vi "PlotCache.vi"(8 "Op":T1(ring), 9 "PlotName":string, 11 "Plot":cluster{"Days":timestamp[], dbl[]}[](graph)) -> (0 "Name":string, 2 "Names":string[](array[string]), 3 "PlotOut":cluster{"Days":timestamp[], dbl[]}[](graph))   [LabVIEW 2017]
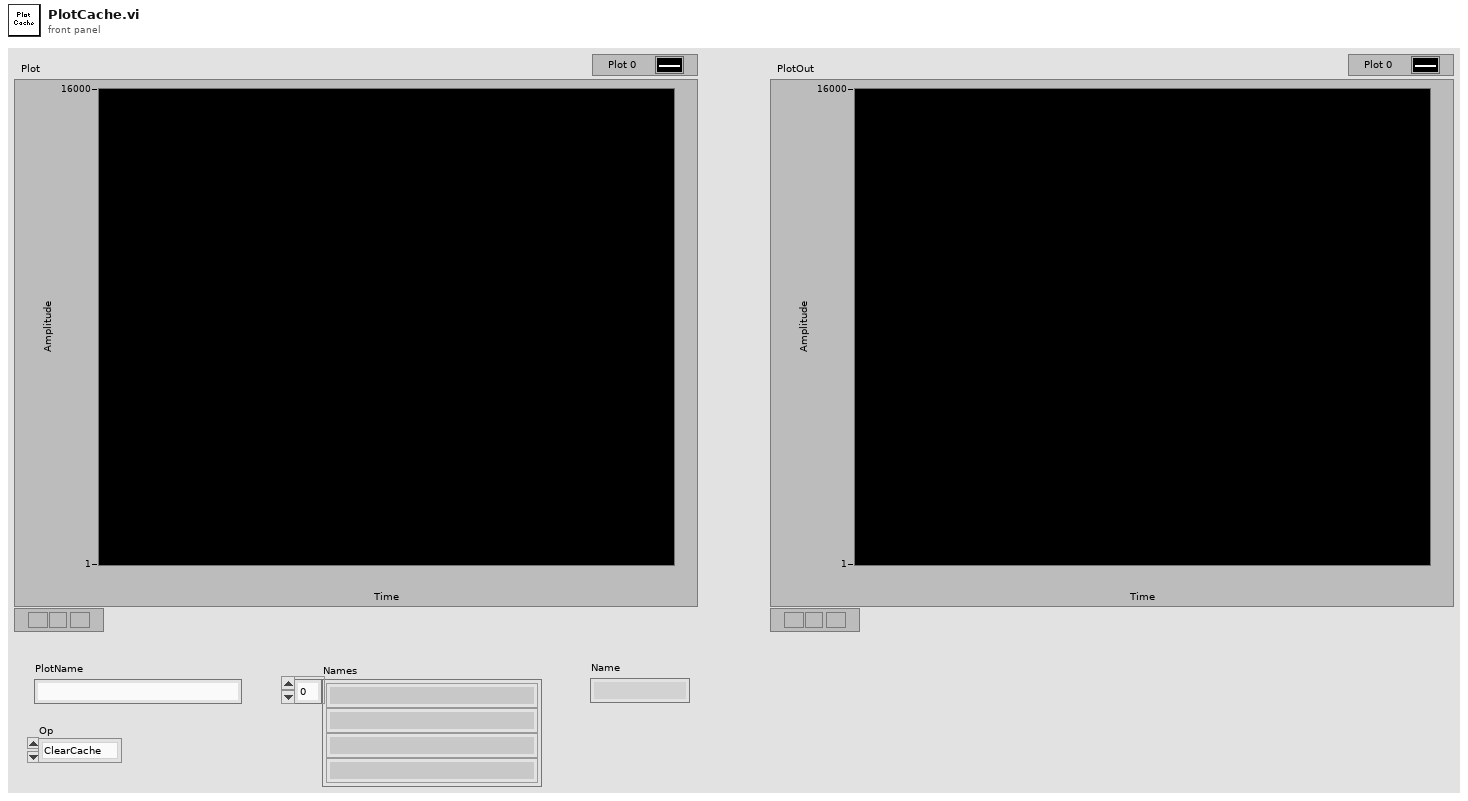
[diagram p1: front panel]
types:
  T1 = enum16{"ClearCache", "AddPlot", "GetPlot", "GetNames", "LastPlot"}
  T2 = cluster{"PlotName":string, "Plot":cluster{"Days":timestamp[], dbl[]}[]}[]
  T3 = cluster{"PlotName":string, "Plot":cluster{"Days":timestamp[], dbl[]}[]}
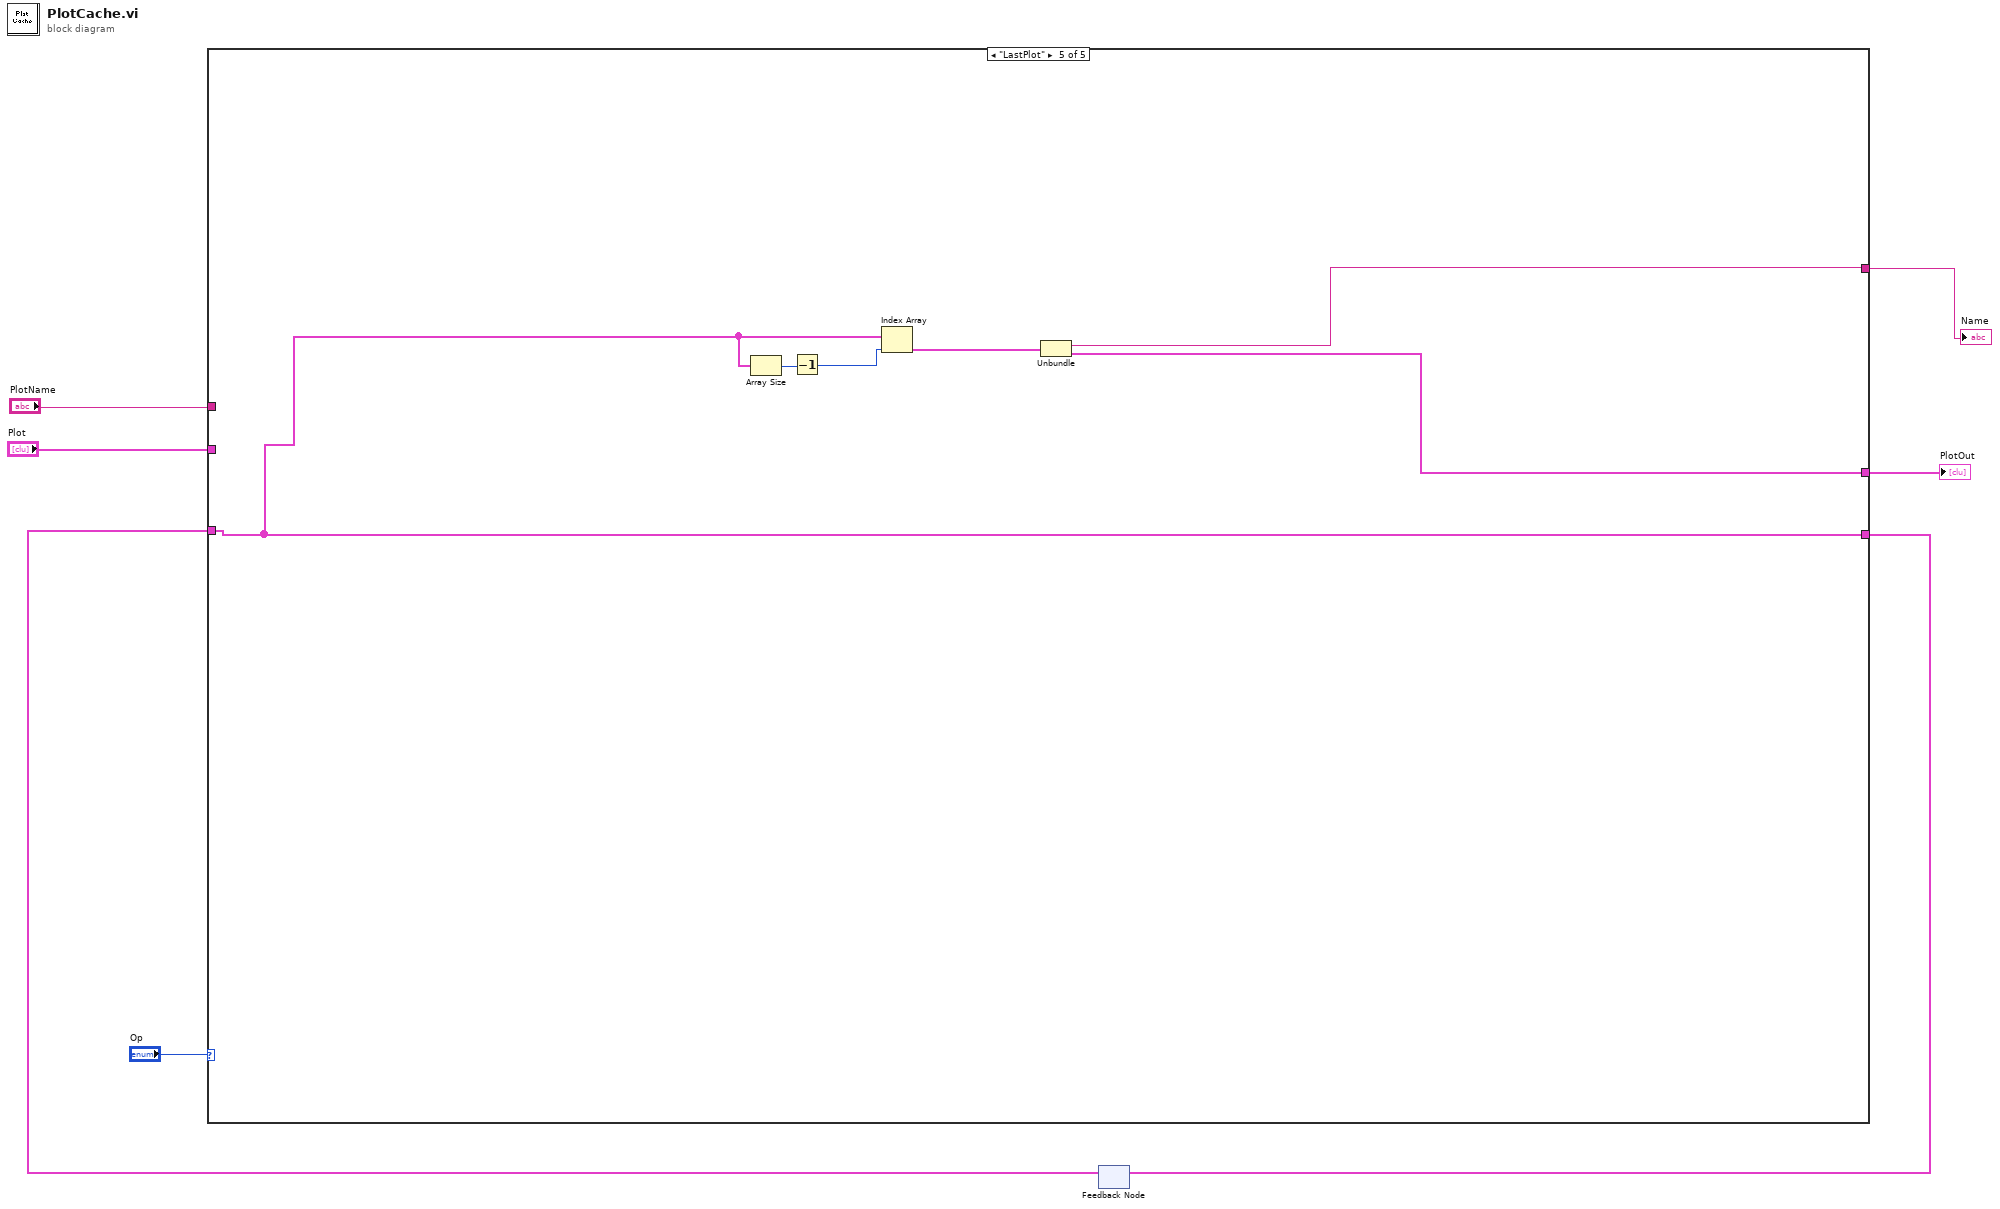
[diagram p0: block diagram]
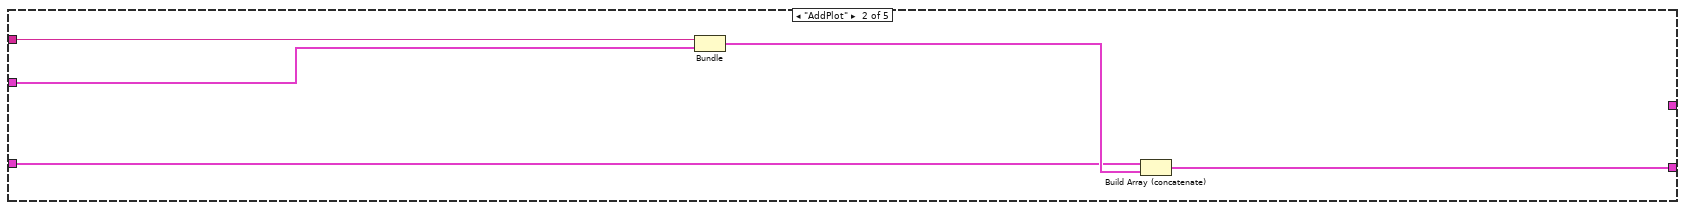
[diagram p3: hidden frame]
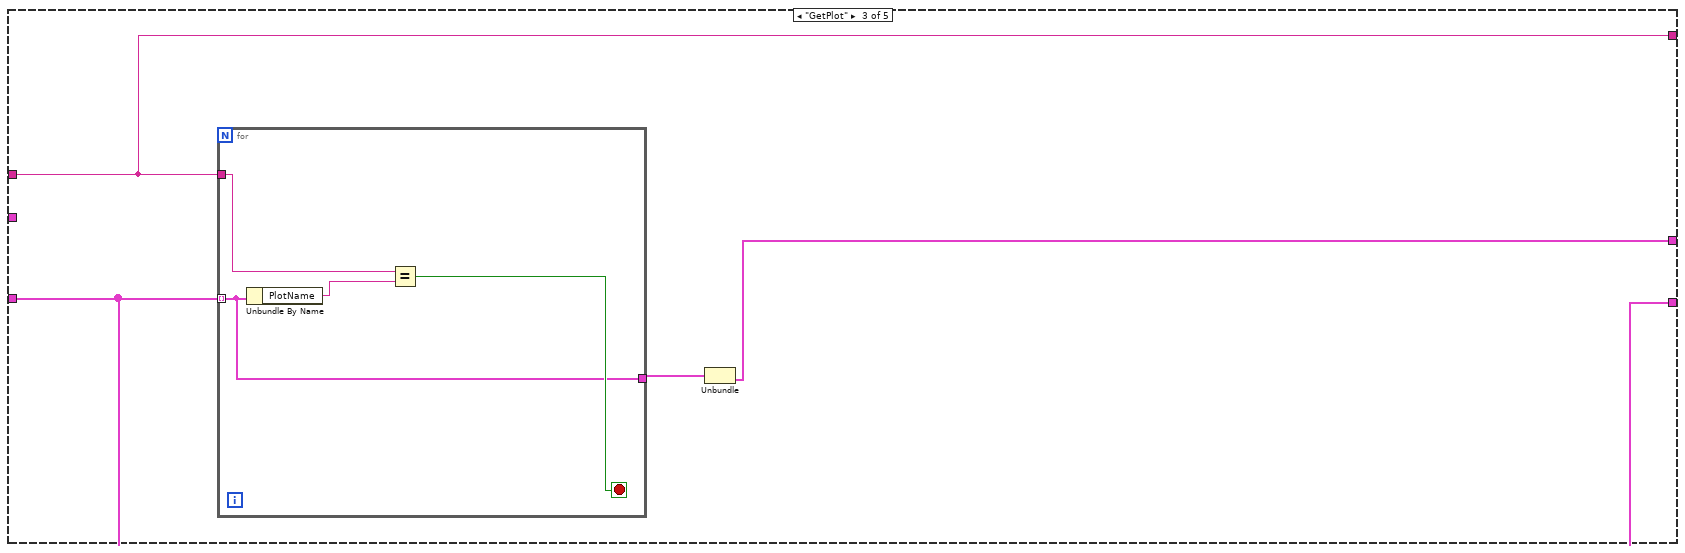
[diagram p4: hidden frame]
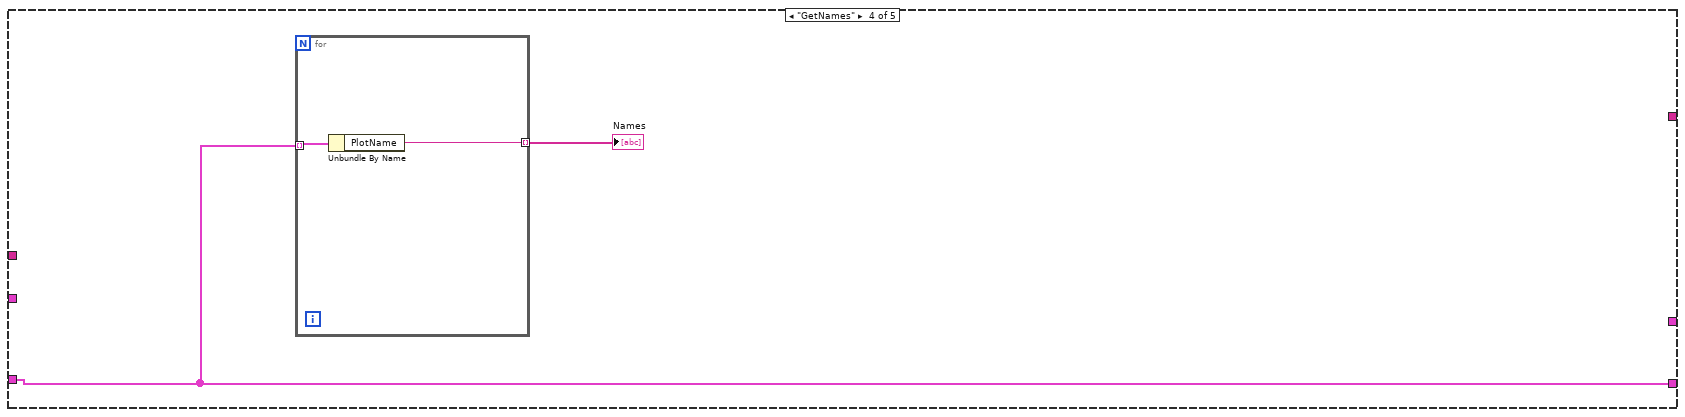
[diagram p5: hidden frame]
diagram:
  n1 = feedback #1() -> (w3:T2)  [unwired: 1 in]
  n2 = case shown="\"LastPlot\"" "Op" {
    tunnel: "Plot" -> [_ w11 _ _ _]
    tunnel: "PlotName" -> [_ w12 w14 _ _]
    tunnel: [_ w9 w16 w22 w28] -> w4
    tunnel: w3 -> [_ w8 w16 w22 w28]
    tunnel: [_ _ w14 _ w26] -> w2
    tunnel: [_ _ w13 _ w25] -> w1
    frame "ClearCache", Default {
    }
    frame "AddPlot" {
      n3 = Bundle("PlotName"=w12, "Plot"=w11) -> (w10:T3)  [unwired: 1 in]
      n4 = Build Array (concatenate)(w8, w10) -> (w9:T2)
    }
    frame "GetPlot" {
      n5 = for {
        tunnel: w16 -> [w17] mode=indexing
        tunnel: w14 -> [w19]
        tunnel: [w17] -> w15
        stop <- w18 stop-if-true
        n6 = Unbundle By Name(w17) -> ("PlotName"=w20:string)
        n7 = Equal?(x=w19, y=w20) -> (x = y?=w18:bool)
      }
      n8 = Unbundle(w15) -> ("Plot"=w13:cluster{"Days":timestamp[], dbl[]}[])  [unwired: 1 out]
    }
    frame "GetNames" {
      n9 = for {
        tunnel: w22 -> [w24] mode=indexing
        tunnel: [w23] -> w21 mode=indexing
        n10 = Unbundle By Name(w24) -> ("PlotName"=w23:string)
      }
      "Names" <- w21
    }
    frame "LastPlot" {
      n11 = Array Size(array=w28) -> (size(s)=w30:i32)
      n12 = Decrement(x=w30) -> (x-1=w29:i32)
      n13 = Index Array(array=w28, index=w29) -> (element=w27:T3)
      n14 = Unbundle(w27) -> ("PlotName"=w26:string, "Plot"=w25:cluster{"Days":timestamp[], dbl[]}[])
    }
  }
  "Name" <- w2
  "PlotOut" <- w1
  n15 = feedback-in #1(w4) -> ()
